vi "Initial State Example - Looping.vi"() -> ()   [LabVIEW 2013]
uses:
  Initial State LabVIEW SDK/Custom Data Types/IS Data Point TypeDef (String).ctl
  Initial State LabVIEW SDK/Data Helpers/IS PolyVI Instance Bool To JSON Cluster .vi
  Initial State LabVIEW SDK/Data Helpers/IS PolyVI Instance String to JSON Cluster.vi
  Initial State LabVIEW SDK/Data Helpers/IS PolyVI Instance DBL To JSON Cluster .vi
panel:
  out "Buffer Size":i32
  in  "stop":bool
  out "Waveform Chart":dbl(graph)=0.6082396240250167
  in  "Bucket Name (Optional)":string="LabVIEW Example Bucket"
  in  "Access Key":string="FakeFakeVj0GLMeSHRkyOEAPFGhzWEmw"
  out "Response Headers":string
  out "Response Body":string
  # "Initial State Streaming LabVIEW Example"
  # "To use this example first create an Initial State account for free at www.initialstate.com. Once created place your access key in the associated field below and hit run."
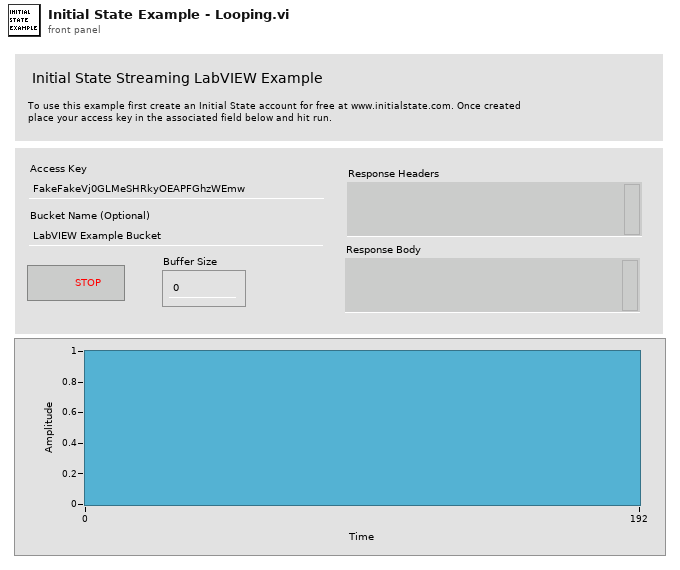
[diagram p1: front panel]
types:
  T1 = typedef "IS Data Point TypeDef (String).ctl" = cluster{"key":string, "value":string, "epoch":dbl}
  T2 = typedef "IS Session.ctl" = cluster{"Access Key":string, "HTTP Client Handle":T3}
  T3 = typedef "LabVIEWHTTPClient.lvlib/ClientHandle.ctl" = refnum<k1>
  T4 = typedef "IS Bucket Session.ctl" = cluster{"Bucket Key":string}
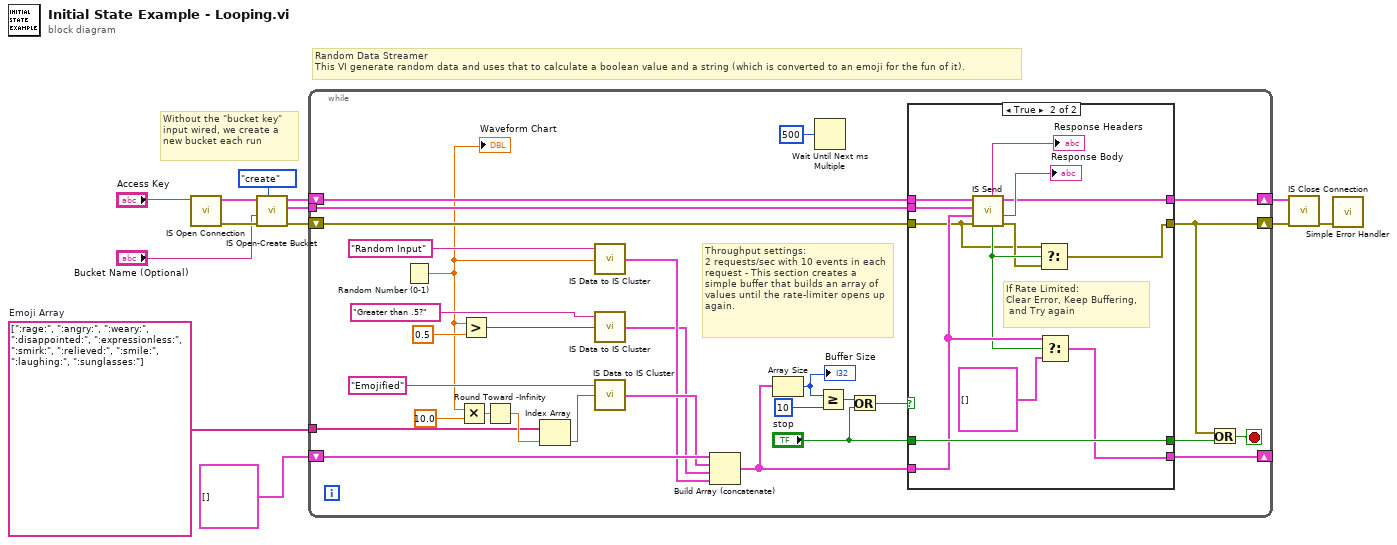
[diagram p0: block diagram]
diagram:
  w4 = string[] [":rage:", ":angry:", ":weary:", ":disappointed:", ":expressionless:", ":smirk:", ":relieved:", ":smile:", ":laughing:", ":sunglasses:"]  # Emoji Array
  # "Without the \"bucket key\" input wired, we create a new bucket each run"
  # "Random Data Streamer\nThis VI generate random data and uses that to calculate a boolean value and a string (which is converted to an emoji for the fun of it)."
  n1 = call "IS Open Connection.vi"("Access Key"="Access Key") -> ("error out"=w11:errorcluster, "IS Session"=w13:T2)  [unwired: 9 in]
  n2 = call "IS Open-Create Bucket.vi"("Operation (0: open)"=enum16{"open", "create"}."create", "error in (no error)"=w11, "Bucket Name (Optional)"="Bucket Name (Optional)", "IS Session In"=w13) -> ("error IO"=w5:errorcluster, "IS Bucket Session"=w8:T4, "IS Session Out"=w7:T2)  [unwired: 5 in]
  n3 = while {
    tunnel: w8 -> [w40]
    shift-right: [w43] -> w3
    shift-left: w7 -> [w42]
    shift-right: [w23] -> w2
    shift-left: w5 -> [w41]
    shift-right: [w38] -> _
    shift-left: T1[] [] -> [w39]
    tunnel: w4 -> [w28]
    stop <- w22 stop-if-true
    # "Throughput settings: \n2 requests/sec with 10 events in each request - This section creates a simple buffer that builds an array of values until the rate-limiter opens up again."
    n4 = Random Number (0-1)() -> (number: 0 to 1=w17:dbl)
    "Waveform Chart" <- w17
    n5 = Multiply(x=w17, y=10.0) -> (x*y=w31:dbl)
    n6 = Greater?(x=w17, y=0.5) -> (0:w16:bool)
    n7 = Round Toward -Infinity(1:w31) -> (0:w29:dbl)
    n8 = Index Array(array=w28, index=w29) -> (element=w15:string)
    n9 = call-poly "IS Data to IS Cluster.vi"("Stream Value"=w17, "Stream Key"="Random Input") -> ("JSON Cluster Array out"=w25:T1[])  [unwired: 3 in]
    n10 = call-poly "IS Data to IS Cluster.vi"("Stream Value"=w16, "Stream Key"="Greater than .5?") -> ("JSON Cluster Array out"=w24:T1[])  [unwired: 3 in]
    n11 = call-poly "IS Data to IS Cluster.vi"("Stream Value"=w15, "Stream Key"="Emojified") -> ("JSON Cluster Array out"=w26:T1[])  [unwired: 3 in]
    n12 = Build Array (concatenate)(w39, w26, w24, w25) -> (w37:T1[])
    n13 = Array Size(array=w37) -> (size(s)=w36:i32)
    "Buffer Size" <- w36
    n14 = Wait Until Next ms Multiple(millisecond multiple=u32 500) -> ()  [unwired: 1 out]
    n15 = Greater Or Equal?(x=w36, y=10) -> (x >= y?=w20:bool)
    n16 = Or(x=w20, y="stop") -> (x .or. y?=w19:bool)
    n17 = case shown="True" w19 {
      tunnel: [w47 w56] -> w43
      tunnel: [w46 w48] -> w23
      tunnel: w42 -> [w47 w60]
      tunnel: w41 -> [w46 w49]
      tunnel: w40 -> [_ w59]
      tunnel: w37 -> [w45 w53]
      tunnel: [w45 w52] -> w38
      tunnel: "stop" -> [w44 w57]
      tunnel: [w44 w57] -> w21
      frame False {
      }
      frame True {
        # "If Rate Limited: \nClear Error, Keep Buffering,\n and Try again"
        n18 = call "IS Send.vi"("error in (no error)"=w49, "JSON Custer Array in"=w53, "IS Bucket Session"=w59, "IS Session in"=w60) -> ("Error out"=w50:errorcluster, "Response Body"=→"Response Body":string, "IS Session out"=w56:T2, "Rate Limit Reached?"=w51:bool, "Response Headers"=→"Response Headers":string)  [unwired: 2 in, 1 out]
        n19 = Select(t=w49, s=w51, f=w50) -> (s? t:f=w48:errorcluster)
        n20 = Select(t=w53, s=w51, f=T1[] []) -> (s? t:f=w52:T1[])
      }
    }
    n21 = Or(x=w23, y=w21) -> (x .or. y?=w22:bool)
  }
  n22 = call "IS Close Connection.vi"("error in (no error)"=w2, "IS Session In"=w3) -> ("error out"=w10:errorcluster)  [unwired: 9 in]
  n23 = call <vilib>:"Simple Error Handler.vi"("error in (no error)"=w10) -> ()  [unwired: 4 in, 5 out]
